vi "Read AC Frequency.vi"(8 "error in (no error)":errorcluster, 11 "VISA resource name":refnum<visa-resource-name>) -> (0 "error out":errorcluster, 2 "AC Frequency":dbl, 3 "VISA resource name out":refnum<visa-resource-name>)   [LabVIEW 2020, in "Library Instrument & Equipement.lvlib" / "Library Multimeter.lvlib" / "RIGOL DM3058.lvlib"]
doc: "Reads and returns a single AC frequency measurement from the instrument.\n\n<B>Note:</B>\nThis VI only applies to RIGOL DM3051 model in measurement function AC Current or AC Volts."
uses:
  RIGOL DM3058.lvlib
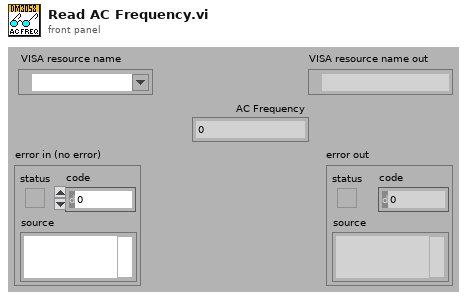
[diagram p1: front panel]
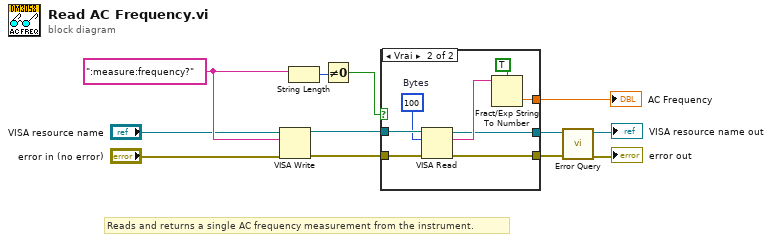
[diagram p0: block diagram]
diagram:
  w3 = ":measure:frequency?" ("multi-line string")
  # "Reads and returns a single AC frequency measurement from the instrument."
  n1 = VISA Write(VISA resource name="VISA resource name", write buffer=w3, error in (no error)="error in (no error)") -> (VISA resource name out=w11:refnum<visa-resource-name>, error out=w12:errorcluster)  [unwired: 1 out]
  n2 = String Length(string=w3) -> (length=w5:i32)
  n3 = Not Equal To 0?(x=w5) -> (x != 0?=w4:bool)
  n4 = case shown="Vrai" w4 {
    tunnel: w12 -> [w13 w22]
    tunnel: w11 -> [w14 w21]
    tunnel: [_ w19] -> w10
    tunnel: [w14 w17] -> w9
    tunnel: [w13 w16] -> w8
    frame False {
    }
    frame True {
      w20 = u32 100  # Bytes
      n5 = VISA Read(VISA resource name=w21, byte count=w20, error in (no error)=w22) -> (VISA resource name out=w17:refnum<visa-resource-name>, read buffer=w18:string, error out=w16:errorcluster)  [unwired: 1 out]
      n6 = Fract/Exp String To Number(use system decimal point (T)=TRUE, string=w18) -> (number=w19:dbl)  [unwired: 3 out]
    }
  }
  "AC Frequency" <- w10
  n7 = call "Error Query.vi"("error in (no error)"=w8, "VISA resource name"=w9) -> ("error out"=→"error out":errorcluster, "VISA resource name out"=→"VISA resource name out":refnum<visa-resource-name>)  [unwired: 8 out]
